vi "Example_Lockin.vi"() -> ()   [LabVIEW 2019]
uses:
  Instrument.Lockin/Instrument.Lockin.lvclass
  Instrument.DAQ/Typedefs/REF.Channel--Cluster--Array.ctl
  Instrument.DAQ/Instrument.DAQ.lvclass
  Instrument.DAQ/Typedefs/REF.Channel--Cluster.ctl
  Instrument.DAQ/Typedefs/AO.Channel.Function--Enum.ctl
  Instrument.DAQ/Typedefs/AO.Channel--Cluster.ctl
  Instrument.DAQ/Typedefs/AO.Channel--Cluster--Array.ctl
panel:
  in  "Channels: AO":T1 {"Phase" format="%.3g"; "Frequency" min=0.0001 max=10000.0 format="%.3g"; "Offset" format="%.3p"; "Amplitude" min=0.0 max=10.0 format="%.3p"}
  in  "Channels: Lockin":T4 {"Roll-Off" min=1; "TC" min=0.0001 format="%#_3p"; "Phase" format="%.3g"; "Frequency" min=0.0001 max=10000.0 format="%.3g"; "Channel" min=1}
  out "Lockin vs time":cluster{timestamp[], dbl[]}(graph)
  out "Lockin vs parameter":cluster{"Y":dbl[], "Y":dbl[]}(graph)
  in  "step":dbl=0.025
  in  "end":dbl=0.1
  in  "start":dbl
  # "Lockin Example: Lockin\nMake Sure Lockin Program is running!"
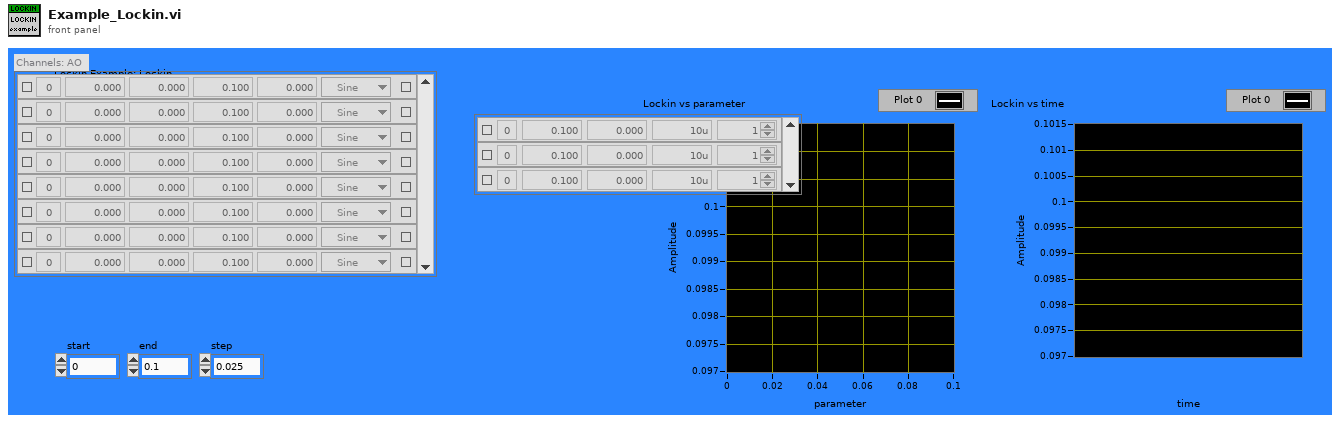
[diagram p1: front panel]
types:
  T1 = typedef "Instrument.Lockin.lvlib/Instrument.DAQ.lvclass/AO.Channel--Cluster--Array.ctl" = T2[]
  T2 = typedef "Instrument.Lockin.lvlib/Instrument.DAQ.lvclass/AO.Channel--Cluster.ctl" = cluster{"Enable?":bool, "Channel":i32, "Amplitude":dbl, "Offset":dbl, "Frequency":dbl, "Phase":dbl, "Function":T3, "Sweeping?":bool}
  T3 = typedef "Instrument.Lockin.lvlib/Instrument.DAQ.lvclass/AO.Channel.Function--Enum.ctl" = enum16{"Sine", "Triangle", "Square"}
  T4 = typedef "Instrument.Lockin.lvlib/Instrument.DAQ.lvclass/REF.Channel--Cluster--Array.ctl" = T5[]
  T5 = typedef "Instrument.Lockin.lvlib/Instrument.DAQ.lvclass/REF.Channel--Cluster.ctl" = cluster{"Enable?":bool, "Channel":i32, "Frequency":dbl, "Phase":dbl, "TC":dbl, "Roll-Off":i32}
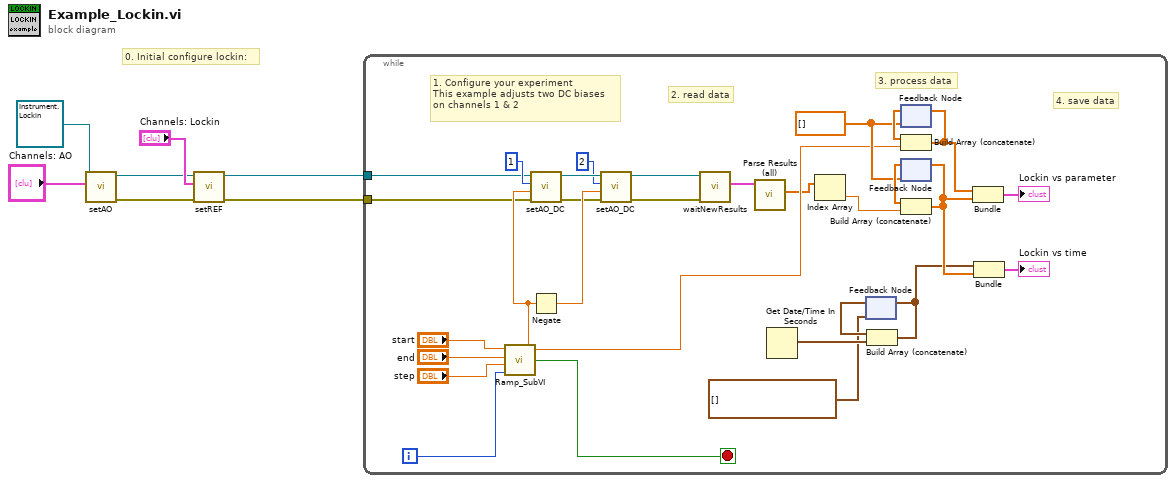
[diagram p0: block diagram]
diagram:
  # "0. Initial configure lockin:"
  n1 = call-dynamic "setAO.vi"("Channels: AO"="Channels: AO", "Instrument.Lockin in"=refnum<class "Instrument.Lockin.lvclass"> refnum) -> ("error out"=w5:errorcluster, "Instrument.Lockin out"=w6:refnum<class "Instrument.Lockin.lvclass">)  [unwired: 8 in]
  n2 = call-dynamic "setREF.vi"("error in (no error)"=w5, "Channels: Lockin in"="Channels: Lockin", "Instrument.Lockin in"=w6) -> ("error out"=w3:errorcluster, "Instrument.Lockin out"=w4:refnum<class "Instrument.Lockin.lvclass">)  [unwired: 7 in]
  n3 = while {
    tunnel: w3 -> [w14]
    tunnel: w4 -> [w13]
    i -> [w33]
    stop <- w36 stop-if-true
    w22 = dbl[] []
    # "4. save data"
    # "3. process data"
    # "2. read data"
    # "1. Configure your experiment\nThis example adjusts two DC biases\non channels 1 & 2"
    n4 = call <userlib>:"Ramp_SubVI.vi"("index"=w33, "step"="step", "end"="end", "start"="start") -> ("Stop?"=w36:bool, "Numeric"=w17:dbl)  [unwired: 1 in]
    n5 = call-dynamic "setAO_DC.vi"("error in (no error)"=w14, "DC (V)"=w17, "AO Channel"=1, "Instrument.Lockin in"=w13) -> ("error out"=w15:errorcluster, "Instrument.Lockin out"=w20:refnum<class "Instrument.Lockin.lvclass">)  [unwired: 6 in]
    n6 = Negate(x=w17) -> (-x=w16:dbl)
    n7 = call-dynamic "setAO_DC.vi"("error in (no error)"=w15, "DC (V)"=w16, "AO Channel"=2, "Instrument.Lockin in"=w20) -> ("error out"=w12:errorcluster, "Instrument.Lockin out"=w11:refnum<class "Instrument.Lockin.lvclass">)  [unwired: 6 in]
    n8 = call-dynamic "waitNewResults.vi"("error in (no error)"=w12, "Instrument.Lockin in"=w11) -> ("Results (Dictionary)"=w10:cluster{"key":string, "value":dbl}[])  [unwired: 7 in, 2 out]
    n9 = call "Parse Results (all).vi"("Results (Dictionary)"=w10) -> ("Data"=w9:dbl[])  [unwired: 7 in, 3 out]
    n10 = Get Date/Time In Seconds() -> (seconds since 1Jan1904=w25:timestamp)
    n11 = Index Array(array=w9) -> (element=w8:dbl)  [unwired: 1 in]
    n12 = feedback #1(timestamp[] []) -> (w23:timestamp[])
    n13 = Build Array (concatenate)(w23, w25) -> (w24:timestamp[])
    n14 = feedback-in #1(w24) -> ()
    n15 = feedback #2(w22) -> (w27:dbl[])
    n16 = Build Array (concatenate)(w27, w17) -> (w26:dbl[])
    n17 = feedback-in #2(w26) -> ()
    n18 = feedback #3(w22) -> (w29:dbl[])
    n19 = Build Array (concatenate)(w29, w8) -> (w28:dbl[])
    n20 = feedback-in #3(w28) -> ()
    n21 = Bundle(w26, w28) -> (→"Lockin vs parameter":cluster{dbl[], dbl[]})  [unwired: 1 in]
    n22 = Bundle(w24, w28) -> (→"Lockin vs time":cluster{timestamp[], dbl[]})  [unwired: 1 in]
  }
